vi "user process.vi"(8 "error in":errorcluster, 11 "Parameters to process":T2) -> (0 "error out":errorcluster, 3 "Results from processing":T1)   [LabVIEW 2014, in "CentralErrorHandler runtime.lvclass"]
uses:
  CentralErrorHandler runtime.lvclass
  parameter user data.ctl
  result user data.ctl
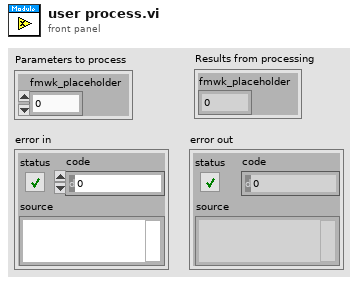
[diagram p1: front panel]
types:
  T1 = typedef "CentralErrorHandler runtime.lvclass/result user data.ctl" = cluster{"fmwk_placeholder":i32}
  T2 = typedef "CentralErrorHandler runtime.lvclass/parameter user data.ctl" = cluster{"fmwk_placeholder":i32}
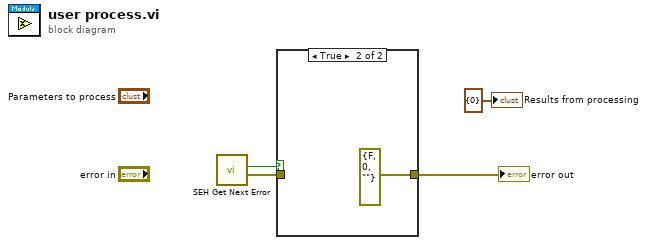
[diagram p0: block diagram]
diagram:
  n1 = call <userlib>:"SEH Get Next Error.vi"() -> ("Transmitted Error"=w2:errorcluster, "Empty?"=w4:bool)  [unwired: 8 in, 2 out]
  n2 = case shown="True" w4 {
    tunnel: [w5 errorcluster {"status"=FALSE, "code"=0, "source"=""} ("error out")] -> w3
    tunnel: w2 -> [w5 _]
    frame False {
    }
    frame True {
    }
  }
  "error out" <- w3
  "Results from processing" <- T1 {"fmwk_placeholder"=0} ("Results from processing")
